vi "New.vi"(8 "error in (no error)":errorcluster, 9 "Resource (None)":string, 10 "Parent":refnum<class "Config Element.lvclass">, 11 "Name":string) -> (0 "error out":errorcluster, 3 "Channel out":refnum<class "Channel Config.lvclass">)   [LabVIEW 2020, in "VolatusConfig.lvlib" / "Channel Config.lvclass"]
uses:
  Channel Config.lvclass
  Channel Config.lvclass/Channel Config.ctl
  lv-cdm/CDM-Config/Config Element/Config Element.lvclass
  lv-cdm/CDM-Config/Value Type.ctl
  lv-cdm/CDM-Config/CDM-Config.lvlib
  VolatusConfig.lvlib
  Meta Type.ctl
  VolatusConfigElement/VolatusConfigElement.lvclass
  C:/dev/lv20CE/relink/lv-volatus/VolatusConfig/VolatusConfigElement/VolatusConfigElement.lvclass
  C:/dev/lv20CE/relink/lv-volatus/VolatusConfig/Channel/Channel Config.lvclass
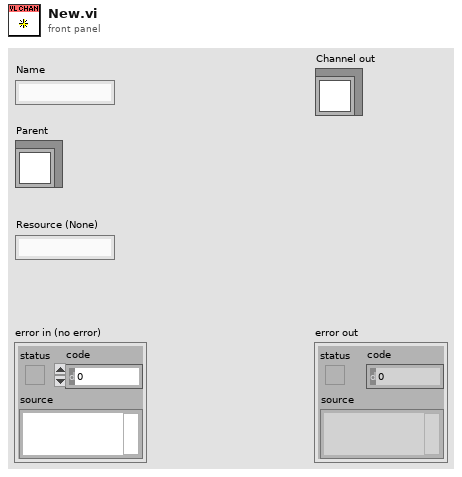
[diagram p1: front panel]
types:
  T1 = typedef "VolatusConfig.lvlib/Meta Type.ctl" = enum16{"UNKNOWN", "VL_System", "VL_Cluster", "VL_Node", "VL_Task", "VL_Group", "VL_Channel", "VL_Task_List", "VL_Scaling", "VL_Sensor", "VL_Sensor_List", "VL_Scale"}
  T2 = typedef "CDM-Config.lvlib/Value Type.ctl" = enum16{"String", "Number", "Bool", "Object", "Array"}
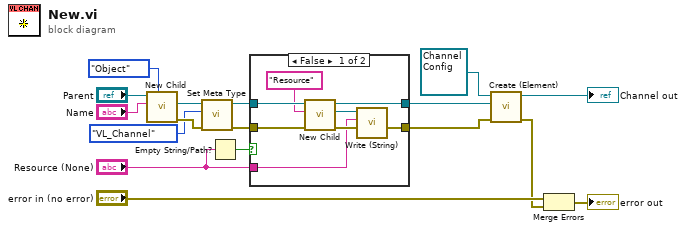
[diagram p0: block diagram]
diagram:
  n1 = call "New Child.vi"("Value Type (Object)"=Value_Type."Object" ("Value Type (String)"), "Child Name"="Name", "Config Element in"="Parent") -> ("error out"=w17:errorcluster, "New Child"=w11:refnum<class "Config Element.lvclass">)  [unwired: 6 in, 1 out]
  n2 = call "Set Meta Type.vi"("error in (no error)"=w17, "Meta Type"=Meta_Type."VL_Channel", "Element In"=w11) -> ("error out"=w8:errorcluster, "Element"=w9:refnum<class "Config Element.lvclass">)  [unwired: 7 in]
  n3 = Empty String/Path?(string/path="Resource (None)") -> (empty?=w7:bool)
  n4 = case shown="False" w7 {
    tunnel: w9 -> [w25 w27]
    tunnel: w8 -> [w24 w26]
    tunnel: "Resource (None)" -> [w20 _]
    tunnel: [w19 w27] -> w4
    tunnel: [w18 w26] -> w3
    frame False {
      n5 = call "New Child.vi"("error in (no error)"=w24, "Child Name"="Resource", "Config Element in"=w25) -> ("error out"=w22:errorcluster, "New Child"=w21:refnum<class "Config Element.lvclass">, "Config Element out"=w19:refnum<class "Config Element.lvclass">)  [unwired: 6 in]
      n6 = call "Write (String).vi"("error in (no error)"=w22, "String Value"=w20, "Config Element in"=w21) -> ("error out"=w18:errorcluster)  [unwired: 7 in, 1 out]
    }
    frame True {
    }
  }
  n7 = call "Create (Element).vi"("error in (no error)"=w3, "Element"=w4, "VolatusConfigElement in"=refnum<class "Channel Config.lvclass"> refnum ("Channel in")) -> ("error out"=w1:errorcluster, "VolatusConfigElement out"=→"Channel out":refnum<class "Channel Config.lvclass">)  [unwired: 7 in]
  n8 = Merge Errors("error in (no error)", w1) -> (→"error out":errorcluster)
